vi "LinearVelocity.vi"(10 "Velocity":dbl, 11 "LineArray":cluster{"X":dbl, "Y":dbl, "OnOff":bool}[](array[cluster])) -> (0 "XY Graph":cluster{"X":dbl, "Y":dbl}[](graph), 2 "Yvelocities":cluster{"Time":dbl, "Velocity":dbl, "Y":dbl}[](array[cluster]), 3 "Xvelocities":cluster{"Time":dbl, "Velocity":dbl, "X":dbl}[](array[cluster]))   [LabVIEW 2012]
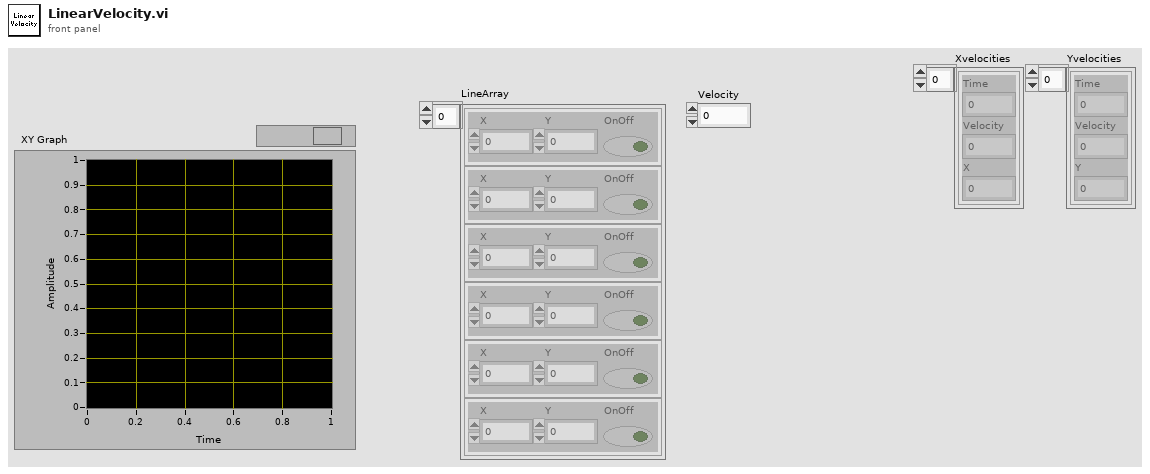
[diagram p1: front panel]
types:
  T1 = cluster{"Time":dbl, "Velocity":dbl, "Position":dbl}
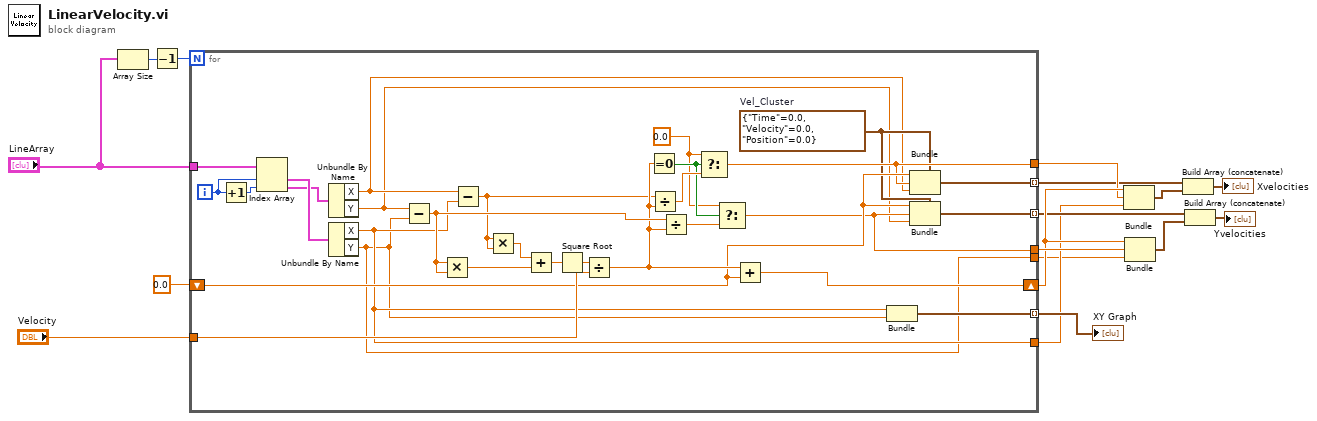
[diagram p0: block diagram]
diagram:
  n1 = Array Size(array="LineArray") -> (size(s)=w17:i32)
  n2 = Decrement(x=w17) -> (x-1=w16:i32)
  n3 = for {
    N: w16 -> [_]
    tunnel: "LineArray" -> [w46]
    tunnel: "Velocity" -> [w41]
    tunnel: [w37] -> w15 mode=indexing
    shift-right: [w30] -> w12
    shift-left: 0.0 -> [w29]
    tunnel: [w28] -> w8 mode=indexing
    tunnel: [w27] -> w10 mode=indexing
    tunnel: [w26] -> w13
    tunnel: [w25] -> w11
    tunnel: [w20] -> w6
    tunnel: [w18] -> w5
    i -> [w43]
    w22 = T1 {"Time"=0.0, "Velocity"=0.0, "Position"=0.0}  # Vel_Cluster
    w32 = 0.0
    n4 = Increment(x=w43) -> (x+1=w44:i32)
    n5 = Index Array(array=w46, index #1=w43, index #2=w44) -> (element #1=w45:cluster{"X":dbl, "Y":dbl, "OnOff":bool}, element #2=w42:cluster{"X":dbl, "Y":dbl, "OnOff":bool})
    n6 = Unbundle By Name(w42) -> ("X"=w21:dbl, "Y"=w19:dbl)
    n7 = Unbundle By Name(w45) -> ("X"=w20:dbl, "Y"=w18:dbl)
    n8 = Subtract(x=w19, y=w18) -> (x-y=w38:dbl)
    n9 = Multiply(x=w38, y=w38) -> (x*y=w39:dbl)
    n10 = Subtract(x=w21, y=w20) -> (x-y=w31:dbl)
    n11 = Multiply(x=w31, y=w31) -> (x*y=w40:dbl)
    n12 = Add(x=w40, y=w39) -> (x+y=w24:dbl)
    n13 = Square Root(x=w24) -> (sqrt(x)=w23:dbl)
    n14 = Divide(x=w23, y=w41) -> (x/y=w35:dbl)
    n15 = Equal To 0?(x=w35) -> (x = 0?=w33:bool)
    n16 = Divide(x=w31, y=w35) -> (x/y=w36:dbl)
    n17 = Divide(x=w38, y=w35) -> (x/y=w34:dbl)
    n18 = Select(t=w32, s=w33, f=w36) -> (s? t:f=w25:dbl)
    n19 = Select(t=w32, s=w33, f=w34) -> (s? t:f=w26:dbl)
    n20 = Add(x=w35, y=w29) -> (x+y=w30:dbl)
    n21 = Bundle("X"=w20, "Y"=w18) -> (w37:cluster{"X":dbl, "Y":dbl})  [unwired: 1 in]
    n22 = Bundle(cluster=w22, "Time"=w29, "Velocity"=w25, "Position"=w21) -> (w27:T1)
    n23 = Bundle(cluster=w22, "Time"=w29, "Velocity"=w26, "Position"=w19) -> (w28:T1)
  }
  "XY Graph" <- w15
  n24 = Bundle(w12, w11, "X"=w6) -> (w9:cluster{dbl, dbl, "X":dbl})  [unwired: 1 in]
  n25 = Bundle(w12, w13, "Y"=w5) -> (w7:cluster{dbl, dbl, "Y":dbl})  [unwired: 1 in]
  n26 = Build Array (concatenate)(w10, w9) -> (→"Xvelocities":cluster{"Time":dbl, "Velocity":dbl, "X":dbl}[])
  n27 = Build Array (concatenate)(w8, w7) -> (→"Yvelocities":cluster{"Time":dbl, "Velocity":dbl, "Y":dbl}[])
